vi "svfa_Linear to dB.vi"(0 "input signal":dbl[](array[numeric]) format="%.2f", 1 "linear/dB desired":enum16{"no change", "linear", "dB"}(ring), 2 "dB reference (desired)":dbl=1.0 format="%.2f", 5 "linear/dB (in)":enum16{"linear", "dB"}(ring), 7 "power/magnitude":enum16{"power", "magnitude"}(ring), 9 "view in":enum16{"rms", "peak", "peak-peak"}(ring), 11 "dB reference":dbl format="%.2f") -> (4 "converted signal":dbl[](array[numeric]) format="%.2f", 6 "linear/dB (out)":enum16{"linear", "dB"}(ring), 8 "power/magnitude (dupl)":enum16{"power", "magnitude"}(ring), 10 "view out":enum16{"rms", "peak", "peak-peak"}(ring), 15 "dB reference (dupl)":dbl format="%.2f")   [LabVIEW 2017]
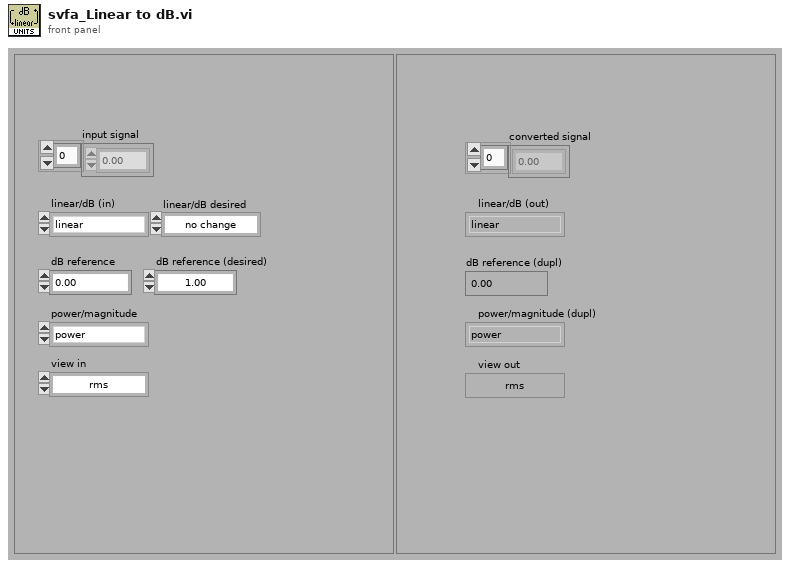
[diagram p1: front panel]
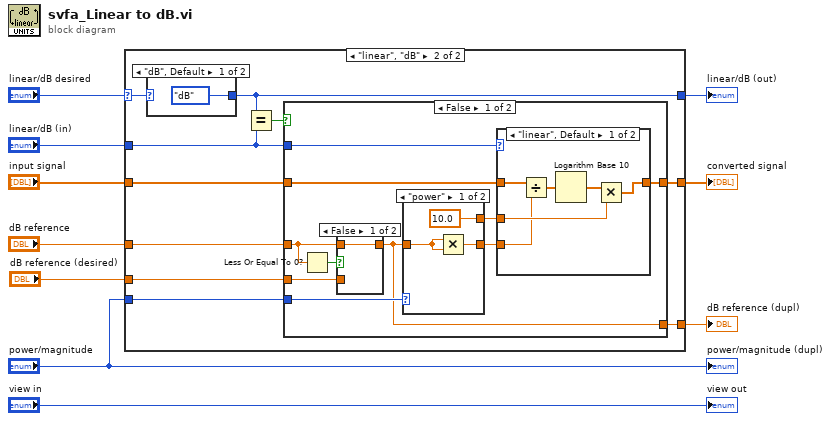
[diagram p0: block diagram]
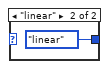
[diagram p3: hidden frame]
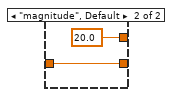
[diagram p4: hidden frame]
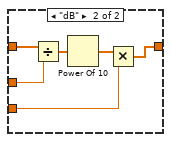
[diagram p6: hidden frame]
diagram:
  n1 = case shown="\"linear\", \"dB\"" "linear/dB desired" {
    selector: "linear/dB desired" -> [_ w16]
    tunnel: [w12 w23] -> w10
    tunnel: "input signal" -> [w12 w22]
    tunnel: "power/magnitude" -> [_ w14]
    tunnel: "dB reference" -> [w11 w21]
    tunnel: [w11 w19] -> w6
    tunnel: "dB reference (desired)" -> [_ w18]
    tunnel: [w13 w15] -> w4
    tunnel: "linear/dB (in)" -> [w13 w17]
    frame "no change", Default {
    }
    frame "linear", "dB" {
      n2 = case shown="\"dB\", Default" w16 {
        tunnel: [enum16{"linear", "dB"}."dB" ("linear/dB (in)") enum16{"linear", "dB"}."linear" ("linear/dB (in)")] -> w15
        frame "dB", Default {
        }
        frame "linear" {
        }
      }
      n3 = Equal?(x=w15, y=w17) -> (x = y?=w20:bool)
      n4 = case shown="False" w20 {
        tunnel: [w34 w56] -> w23
        tunnel: w22 -> [w35 w56]
        tunnel: w17 -> [w33 _]
        tunnel: w21 -> [w27 w55]
        tunnel: [w26 w55] -> w19
        tunnel: w18 -> [w31 _]
        tunnel: w14 -> [w30 _]
        frame False {
          n5 = Less Or Equal To 0?(x=w27) -> (x <= 0?=w32:bool)
          n6 = case shown="False" w32 {
            tunnel: [w41 w42] -> w26
            tunnel: w31 -> [_ w42]
            tunnel: w27 -> [w41 _]
            frame False {
            }
            frame True {
            }
          }
          n7 = case shown="\"power\"" w30 {
            tunnel: [10.0 20.0] -> w28
            tunnel: w26 -> [w37 w39]
            tunnel: [w36 w39] -> w29
            frame "power" {
              n8 = Multiply(x=w37, y=w37) -> (x*y=w36:dbl)
            }
            frame "magnitude", Default {
            }
          }
          n9 = case shown="\"linear\", Default" w33 {
            tunnel: [w45 w51] -> w34
            tunnel: w35 -> [w48 w52]
            tunnel: w29 -> [w43 w49]
            tunnel: w28 -> [w44 w50]
            frame "linear", Default {
              n10 = Divide(x=w48, y=w43) -> (x/y=w47:dbl[])
              n11 = Logarithm Base 10(1:w47) -> (0:w46:dbl[])
              n12 = Multiply(x=w46, y=w44) -> (x*y=w45:dbl[])
            }
            frame "dB" {
              n13 = Divide(x=w52, y=w50) -> (x/y=w53:dbl[])
              n14 = Power Of 10(x=w53) -> (10^x=w54:dbl[])
              n15 = Multiply(x=w54, y=w49) -> (x*y=w51:dbl[])
            }
          }
        }
        frame True {
        }
      }
    }
  }
  "converted signal" <- w10
  "linear/dB (out)" <- w4
  "dB reference (dupl)" <- w6
  "power/magnitude (dupl)" <- "power/magnitude"
  "view out" <- "view in"
